vi "Game LaunchPad.vi"() -> ()   [LabVIEW 2011]
uses:
  <vilib>/Utility/miscctls.llb/LVPositionTypeDef.ctl
panel:
  out "life":dbl
  out "showLifeScoreString":string="Life:      Score:"
  out "showTimeString":string="Time:"
  in  "start":bool
  in  "retry":bool
  out "fish":dbl
  out "time":dbl
  in  "stop":bool
  in  "stop 3":bool
  in  "stop 2":bool
  in  "WindowsMediaPlayer 3":refnum<k7>(container)
  in  "WindowsMediaPlayer 2":refnum<k7>(container)
  in  "WindowsMediaPlayer":refnum<k7>(container)
  out "cat sad picture":picture
  out "cat eat picture":picture
  out "win picture":picture
  out "start picture":picture
  out "badfish Array":picture[][](array[picture])
  out "cat picture":picture
  out "cat position[0-9] 2":dbl
  out "carsh? 2":bool
  out "carsh?":bool
  out "cat position[0-9]":dbl
  out "Fish Array":picture[][](array[picture])
  out "CurrentPath":path
  out "background picture":picture
  # "1"
  # "10"
  # "1"
  # "10"
  # "1"
  # "10"
  # "1"
  # "10"
  # "1"
  # "10"
  # "1"
  # "10"
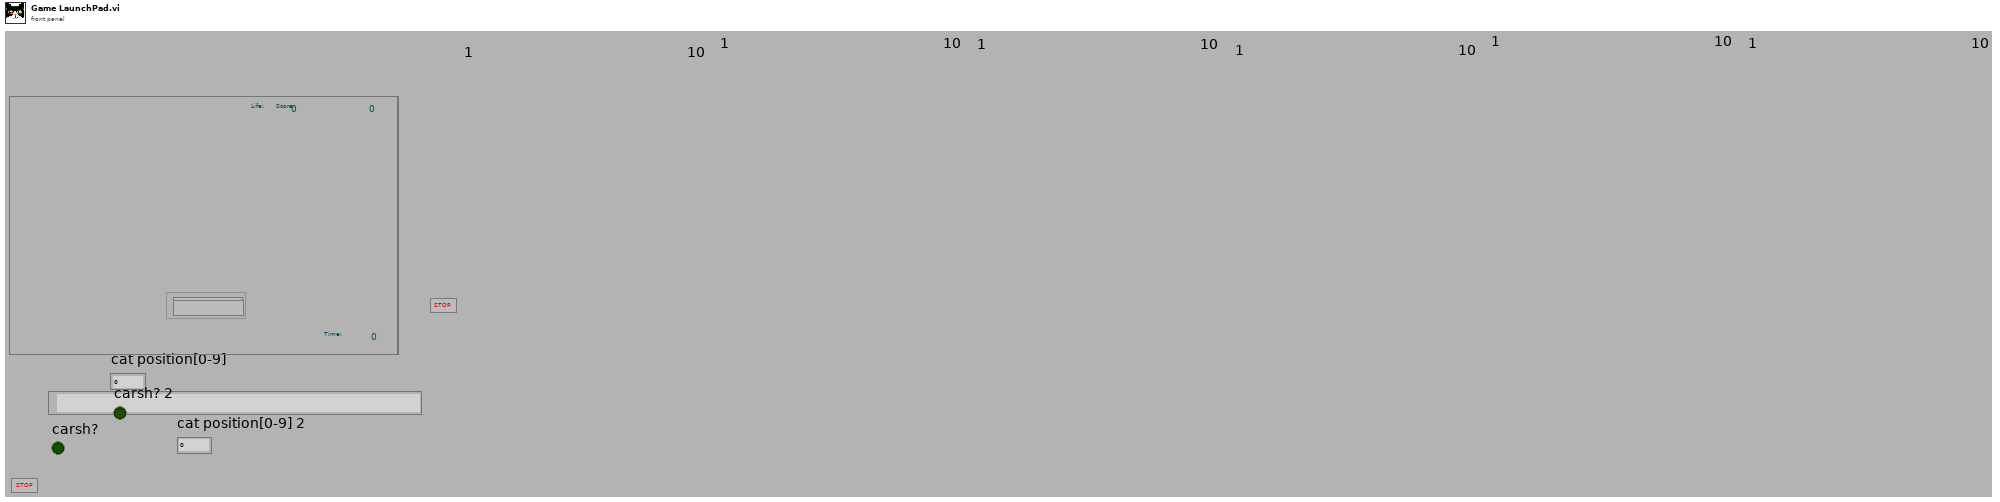
[diagram p1: front panel]
types:
  T1 = enum8{"Enabled", "Disabled", "Disabled and Grayed Out"}
  T2 = typedef "LVPositionTypeDef.ctl" = cluster{"Left":i32, "Top":i32}
  T3 = typedef "imagedata.ctl" = cluster{"image type":i32, "image depth":i32, "image":u8[], "mask":u8[], "colors":u32[], "Rectangle":cluster{"left":i16, "top":i16, "right":i16, "bottom":i16}}
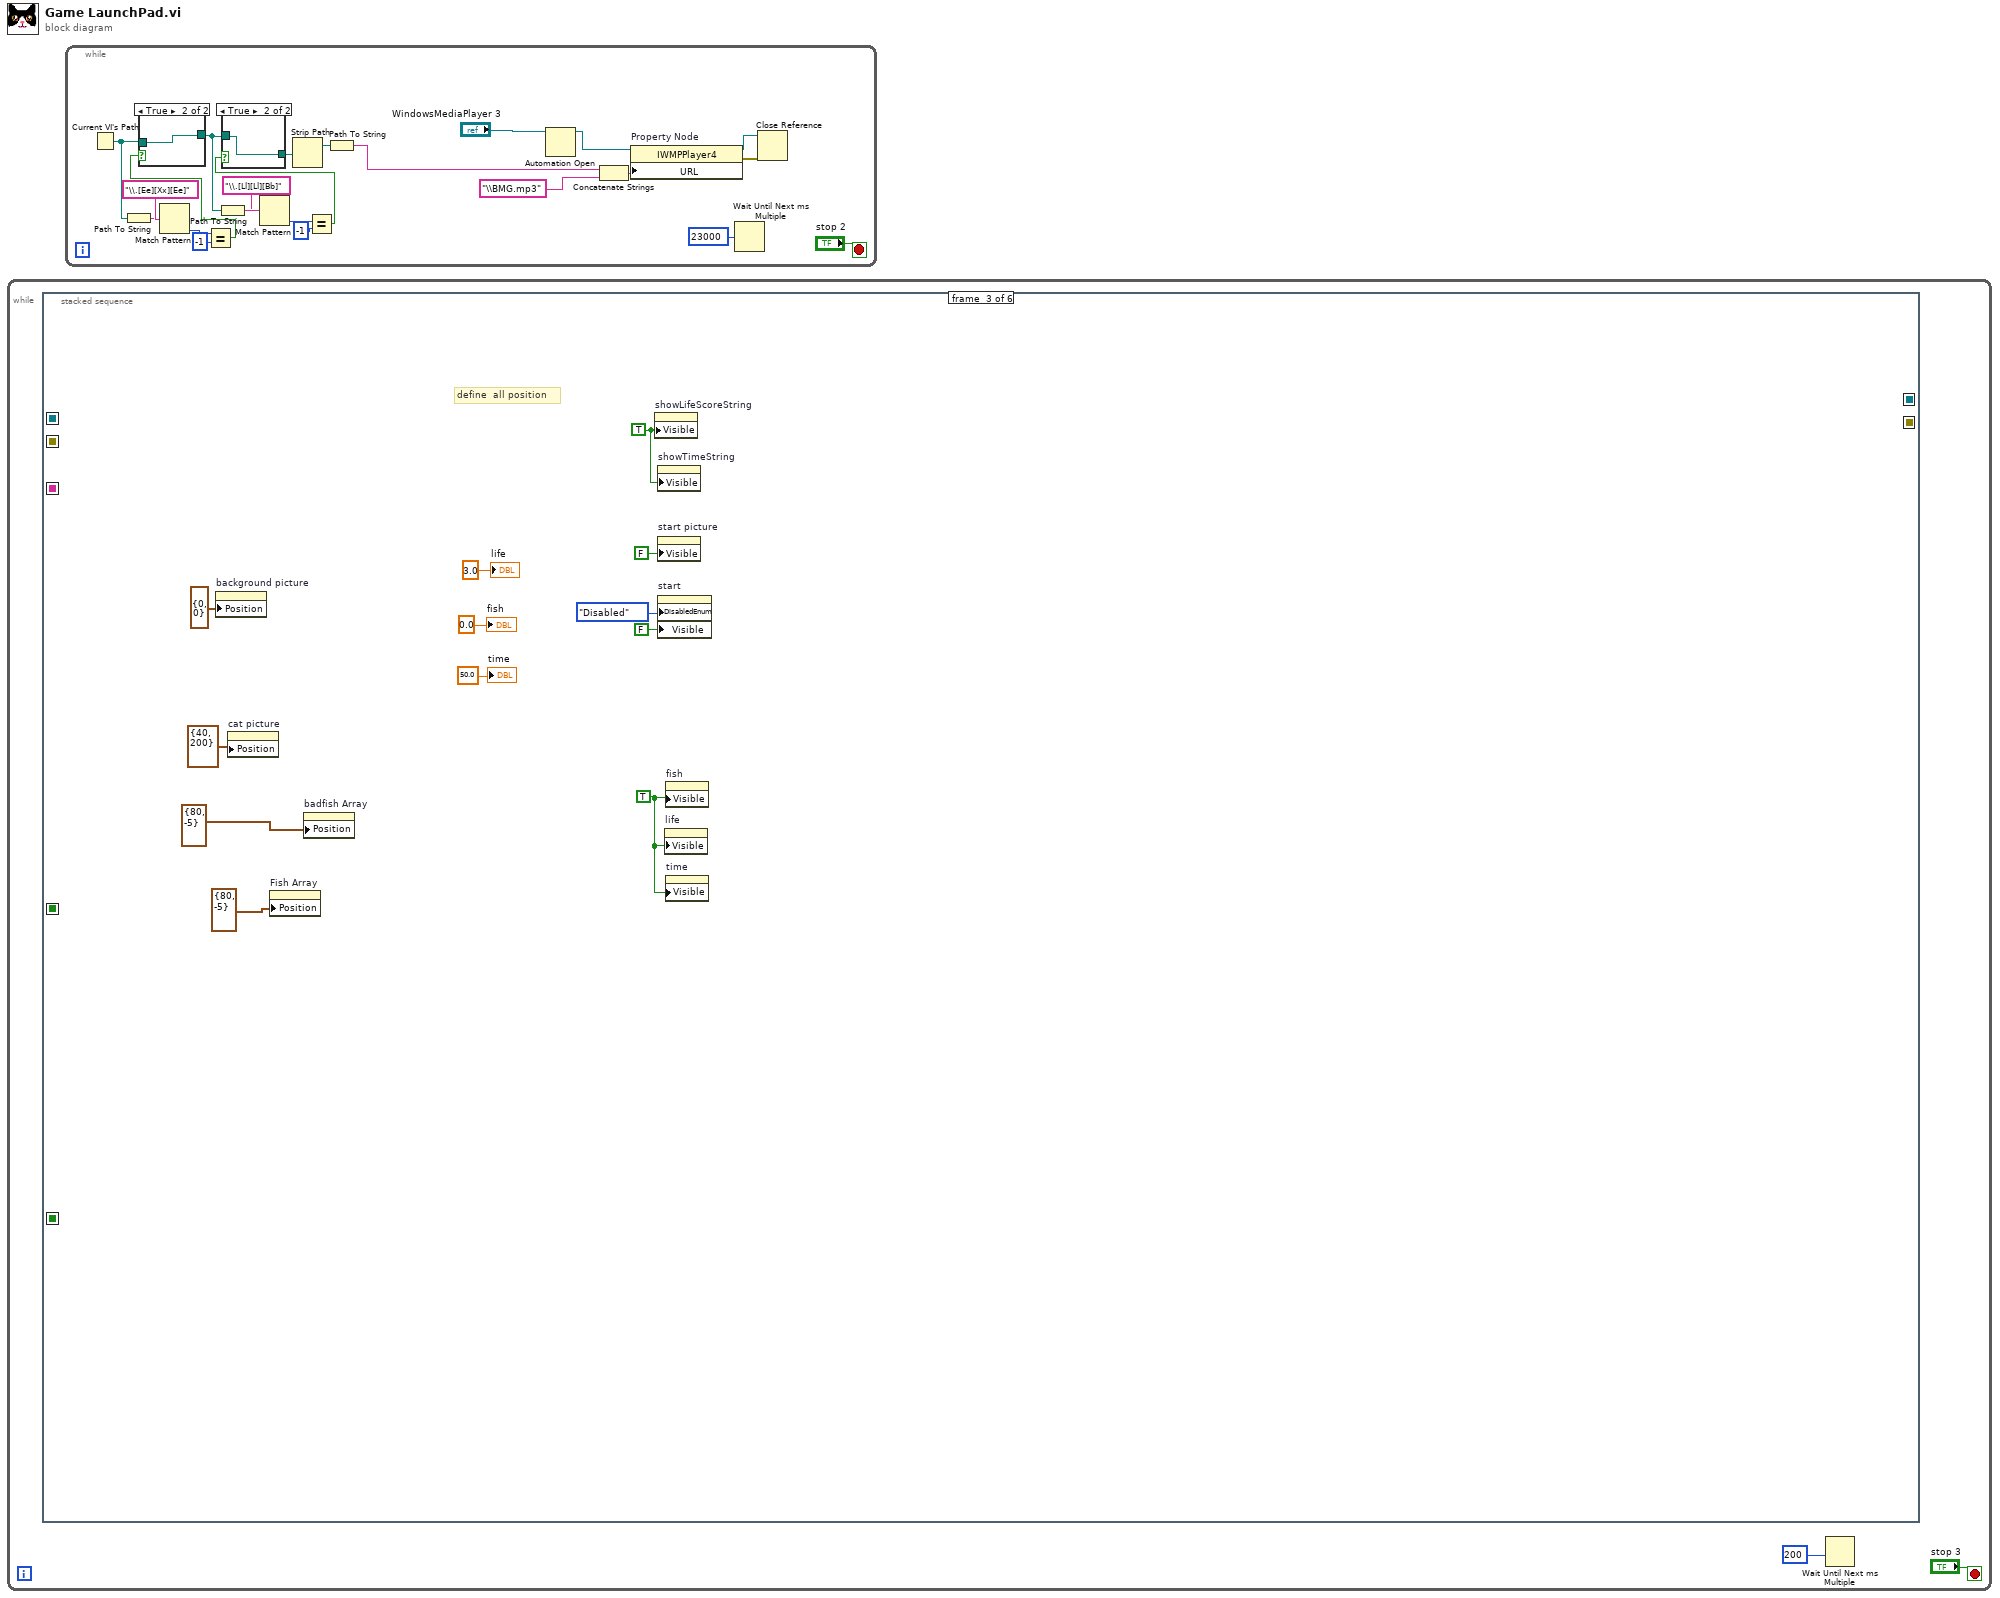
[diagram p0: block diagram]
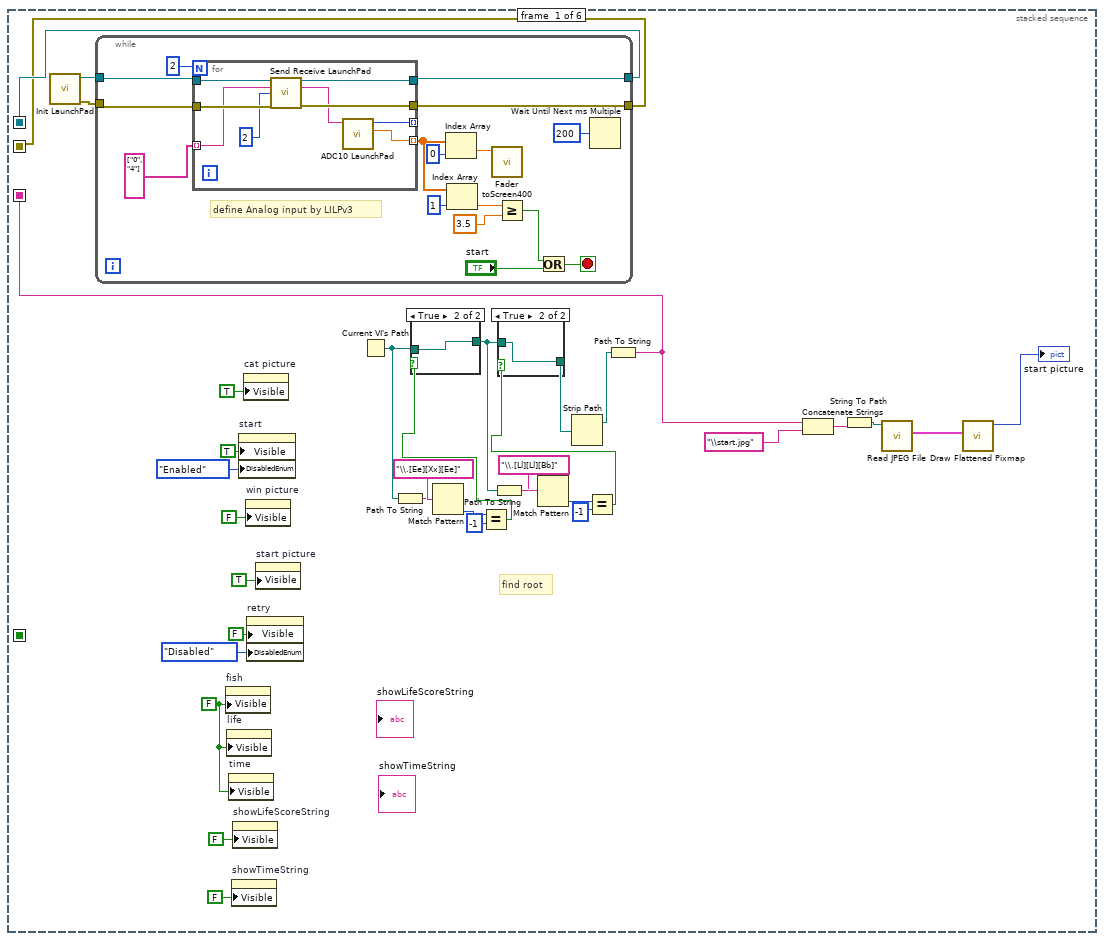
[diagram p2: hidden frame]
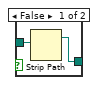
[diagram p3: hidden frame]
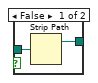
[diagram p4: hidden frame]
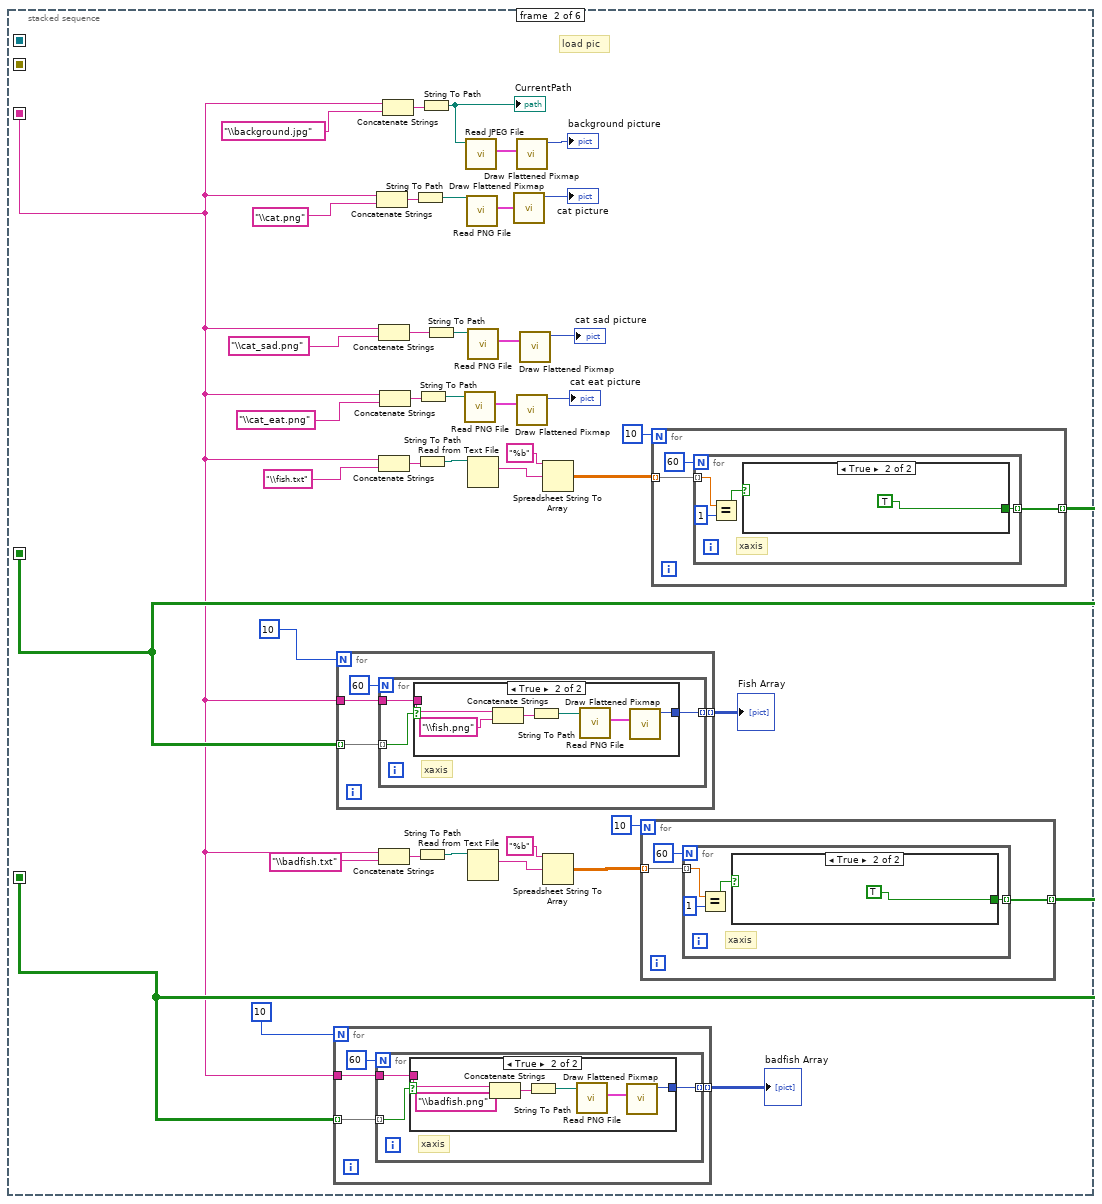
[diagram p5: hidden frame]
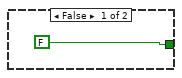
[diagram p6: hidden frame]
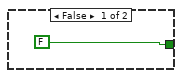
[diagram p7: hidden frame]
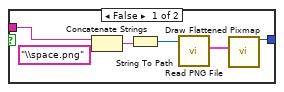
[diagram p8: hidden frame]
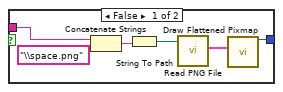
[diagram p9: hidden frame]
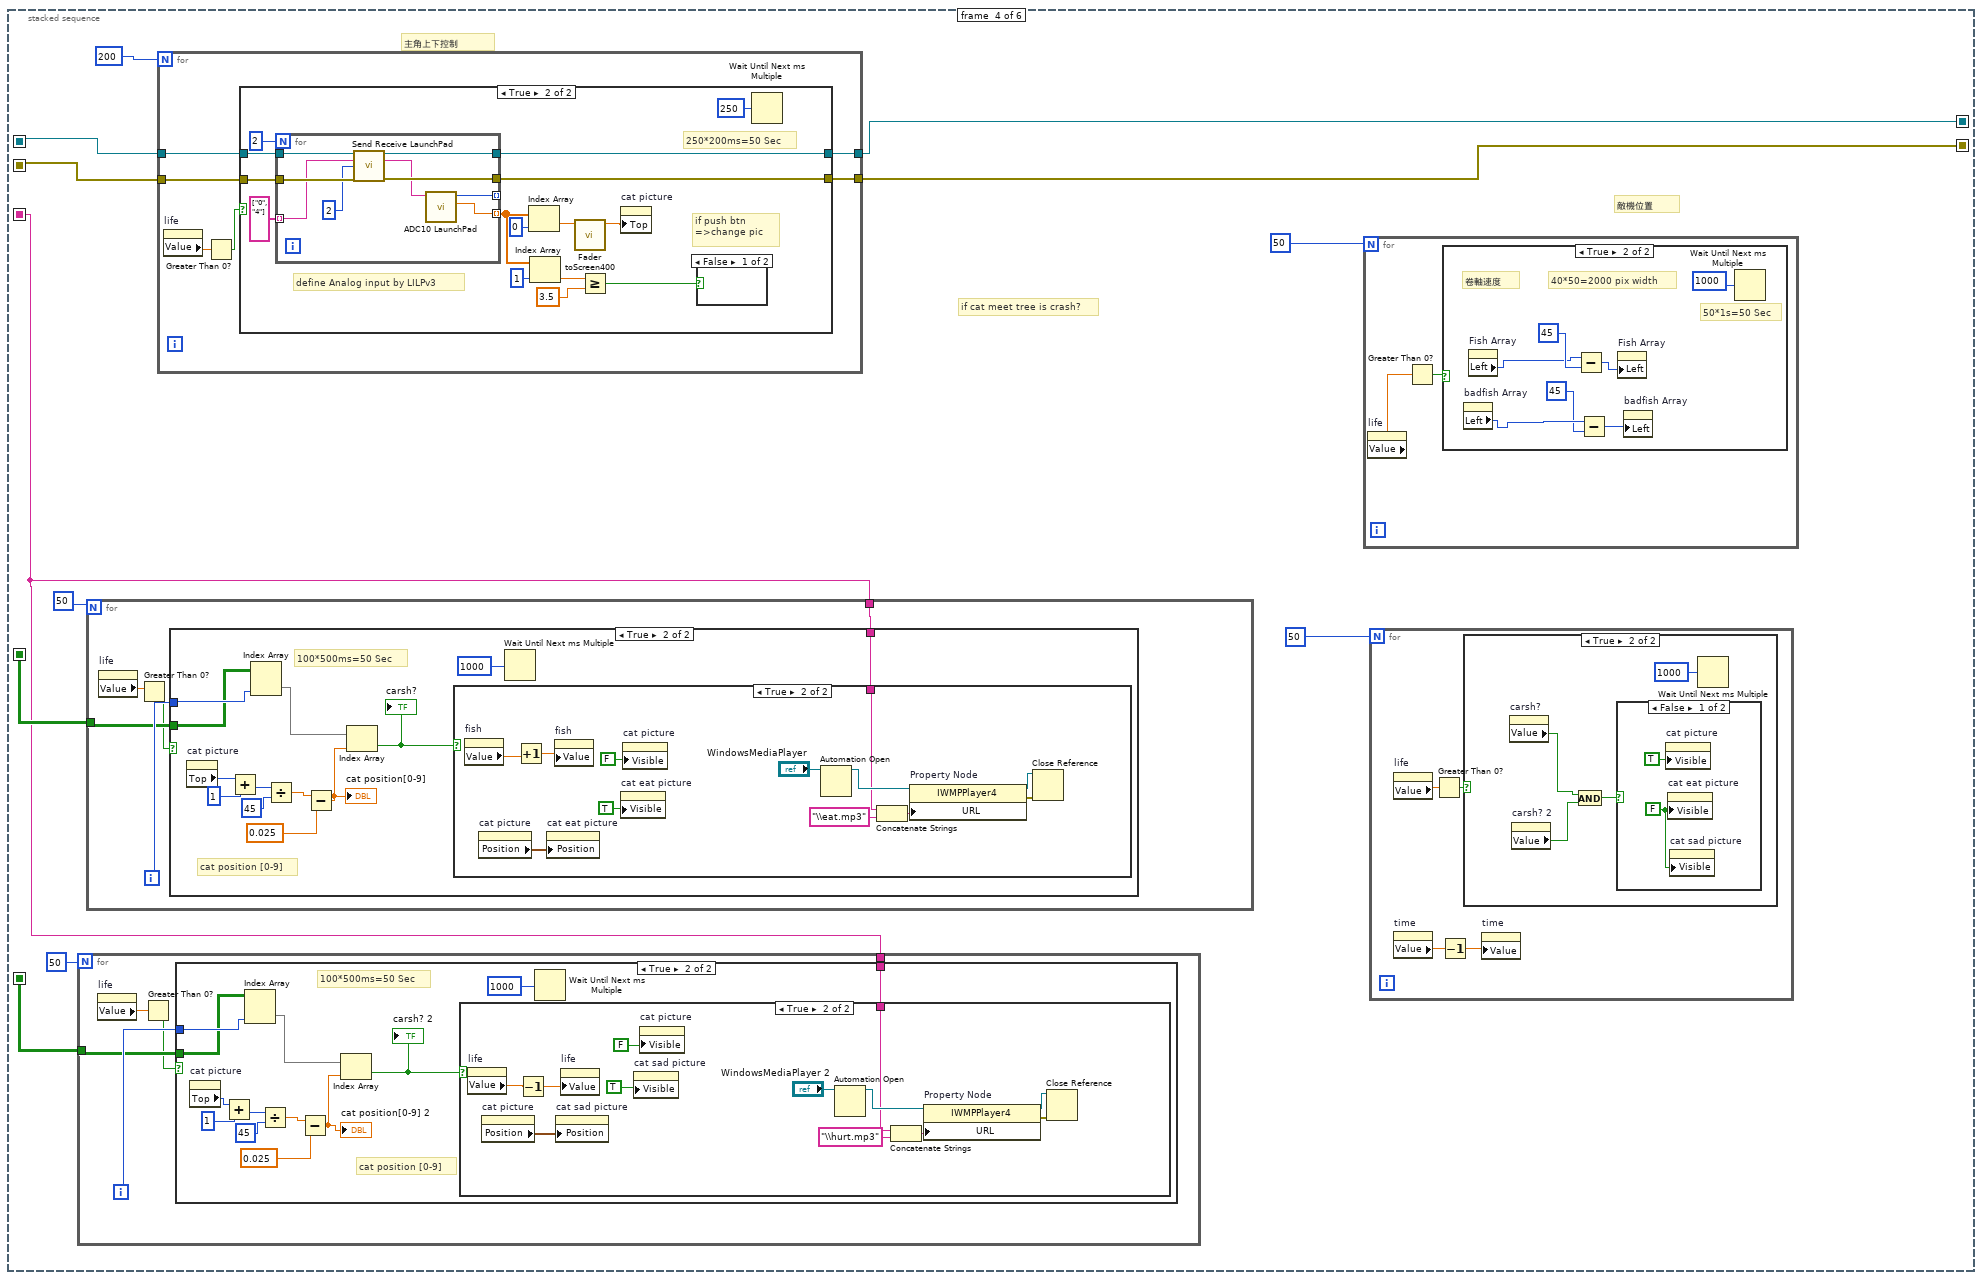
[diagram p10: hidden frame]
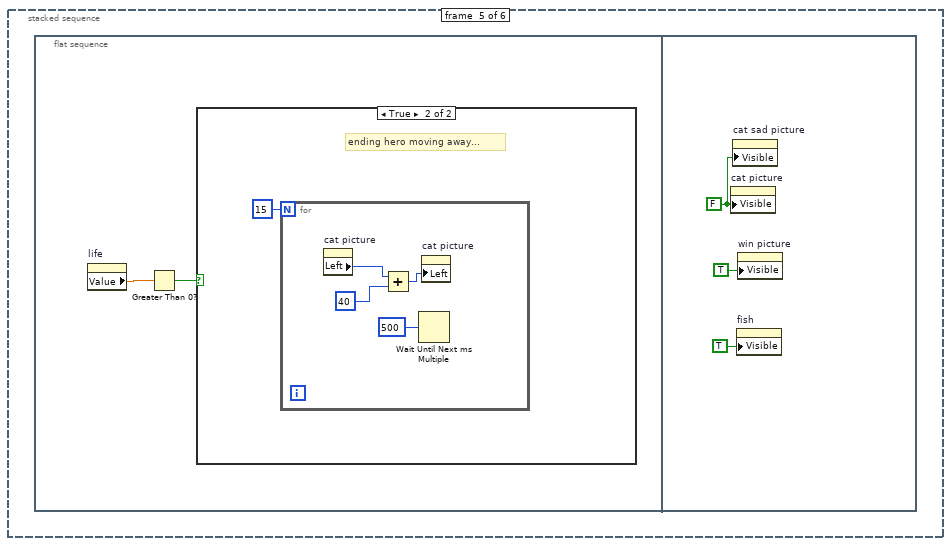
[diagram p20: hidden frame]
diagram:
  n1 = while {
    stop <- "stop 3" stop-if-true
    n2 = stacked-sequence {
      seq-local: [_ w76 _ _ _ _] -> [_ _ _ w184 _ _]
      seq-local: [_ w75 _ _ _ _] -> [_ _ _ w183 _ _]
      seq-local: [w13 _ _ _ _ _] -> [_ w69 _ w179 _ w315]
      seq-local: [w15 _ _ _ _ _] -> [_ _ _ w182 _ _]
      seq-local: [w14 _ _ _ _ _] -> [_ _ _ w181 _ _]
      seq-local: [_ _ _ w178 _ _] -> [_ _ _ _ _ w314]
      seq-local: [_ _ _ w177 _ _] -> [_ _ _ _ _ w313]
      frame #0 {
        w5 = FALSE ("Visible")
        # "find root"
        n3 = call "Init LaunchPad.vi"() -> ("error out"=w16:errorcluster, "VISA resource name out"=w17:refnum<visa-resource-name>)  [unwired: 10 in]
        n4 = while {
          tunnel: w17 -> [w44]
          tunnel: w16 -> [w43]
          tunnel: [w38] -> w15
          tunnel: [w37] -> w14
          stop <- w39 stop-if-true
          # "define Analog input by LILPv3"
          n5 = for {
            N: 2 -> [_]
            tunnel: w44 -> [w61]
            tunnel: [w60] -> w38
            tunnel: [w59] -> w37
            tunnel: w43 -> [w58]
            tunnel: string[] ["0", "4"] -> [w56] mode=indexing
            tunnel: [w54] -> _ mode=indexing
            tunnel: [w53] -> w48 mode=indexing
            n6 = call "Send Receive LaunchPad.vi"("VISA resource"=w61, "write buffer"=w56, "Bytes To Read (0)"=u8 2, "error in"=w58) -> ("VISA resource 2"=w60:refnum<visa-resource-name>, "Read Buffer"=w55:string, "error out"=w59:errorcluster)  [unwired: 9 in]
            n7 = call "ADC10 LaunchPad.vi"("string"=w55) -> ("ADC10 (Volt)"=w53:dbl, "ADCvalue"=w54:u16)  [unwired: 9 in]
          }
          n8 = Index Array(array=w48, index=0) -> (element=w47:dbl)
          n9 = Index Array(array=w48, index=1) -> (element=w45:dbl)
          n10 = call "Fader toScreen400.vi"("Numeric"=w47) -> ()  [unwired: 10 in, 1 out]
          n11 = Greater Or Equal?(x=w45, y=3.5) -> (x >= y?=w41:bool)
          n12 = Or(x=w41, y="start") -> (x .or. y?=w39:bool)
          n13 = Wait Until Next ms Multiple(millisecond multiple=u32 200) -> ()  [unwired: 1 out]
        }
        n14 = property on="fish" class="DigNum (strict)"("Visible"=w5) -> ()  [unwired: 2 in, 2 out]
        n15 = property on="life" class="DigNum (strict)"("Visible"=w5) -> ()  [unwired: 2 in, 2 out]
        n16 = property on="time" class="DigNum (strict)"("Visible"=w5) -> ()  [unwired: 2 in, 2 out]
        n17 = property on="showTimeString" class="Str"("Visible"=FALSE) -> ()  [unwired: 2 in, 2 out]
        n18 = property on="showLifeScoreString" class="Str"("Visible"=FALSE) -> ()  [unwired: 2 in, 2 out]
        n19 = property on="start" class="Bool"("Visible"=TRUE, "DisabledEnum"=T1."Enabled" ("Disabled")) -> ()  [unwired: 2 in, 2 out]
        n20 = property on="cat picture" class="Pict"("Visible"=TRUE) -> ()  [unwired: 2 in, 2 out]
        n21 = property on="win picture" class="Pict"("Visible"=FALSE) -> ()  [unwired: 2 in, 2 out]
        n22 = property on="retry" class="Bool"("Visible"=FALSE, "DisabledEnum"=T1."Disabled" ("Disabled")) -> ()  [unwired: 2 in, 2 out]
        n23 = property on="start picture" class="Pict"("Visible"=TRUE) -> ()  [unwired: 2 in, 2 out]
        n24 = Current VI's Path() -> (path=w27:path)
        n25 = Path To String(path=w27) -> (string=w26:string)
        n26 = Match Pattern(string=w26, regular expression="\\.[Ee][Xx][Ee]") -> (offset past match=w24:i32)  [unwired: 1 in, 3 out]
        n27 = Equal?(x=w24, y=-1) -> (x = y?=w36:bool)
        n28 = case shown="True" w36 {
          tunnel: [w65 w67] -> w33
          tunnel: w27 -> [w66 w67]
          frame False {
            n29 = Strip Path(path=w66) -> (stripped path=w65:path)  [unwired: 1 out]
          }
          frame True {
          }
        }
        n30 = Path To String(path=w33) -> (string=w30:string)
        n31 = Match Pattern(string=w30, regular expression="\\.[Ll][Ll][Bb]") -> (offset past match=w32:i32)  [unwired: 1 in, 3 out]
        n32 = Equal?(x=w32, y=-1) -> (x = y?=w35:bool)
        n33 = case shown="True" w35 {
          tunnel: [w62 w64] -> w34
          tunnel: w33 -> [w63 w64]
          frame False {
            n34 = Strip Path(path=w63) -> (stripped path=w62:path)  [unwired: 1 out]
          }
          frame True {
          }
        }
        n35 = Strip Path(path=w34) -> (stripped path=w23:path)  [unwired: 1 out]
        n36 = Path To String(path=w23) -> (string=w13:string)
        n37 = Concatenate Strings(w13, "\\start.jpg") -> (w19:string)
        n38 = String To Path(string=w19) -> (path=w18:path)
        n39 = call <vilib>:"Read JPEG File.vi"("path to JPEG file"=w18) -> ("image data"=w21:T3)  [unwired: 8 in, 2 out]
        n40 = call <vilib>:"Draw Flattened Pixmap.vi"("image data"=w21) -> ("new picture"=→"start picture":picture)  [unwired: 8 in]
      }
      frame #1 {
        # "load pic"
        n41 = Concatenate Strings(w69, "\\cat.png") -> (w103:string)
        n42 = Concatenate Strings(w69, "\\cat_sad.png") -> (w74:string)
        n43 = Concatenate Strings(w69, "\\fish.txt") -> (w89:string)
        n44 = Concatenate Strings(w69, "\\badfish.txt") -> (w82:string)
        n45 = Concatenate Strings(w69, "\\cat_eat.png") -> (w100:string)
        n46 = Concatenate Strings(w69, "\\background.jpg") -> (w105:string)
        n47 = String To Path(string=w103) -> (path=w97:path)
        n48 = String To Path(string=w89) -> (path=w88:path)
        n49 = String To Path(string=w82) -> (path=w81:path)
        n50 = String To Path(string=w100) -> (path=w95:path)
        n51 = String To Path(string=w105) -> (path=w104:path)
        "CurrentPath" <- w104
        n52 = String To Path(string=w74) -> (path=w71:path)
        n53 = call <vilib>:"Read PNG File.vi"("path to PNG file"=w95) -> ("image data"=w94:T3)  [unwired: 8 in, 2 out]
        n54 = call <vilib>:"Read JPEG File.vi"("path to JPEG file"=w104) -> ("image data"=w107:T3)  [unwired: 8 in, 2 out]
        n55 = call <vilib>:"Read PNG File.vi"("path to PNG file"=w97) -> ("image data"=w96:T3)  [unwired: 8 in, 2 out]
        n56 = call <vilib>:"Read PNG File.vi"("path to PNG file"=w71) -> ("image data"=w70:T3)  [unwired: 8 in, 2 out]
        n57 = Read from Text File(file (use dialog)=w88) -> (text=w87:string)  [unwired: 3 in, 3 out]
        n58 = Read from Text File(file (use dialog)=w81) -> (text=w80:string)  [unwired: 3 in, 3 out]
        n59 = call <vilib>:"Draw Flattened Pixmap.vi"("image data"=w96) -> ("new picture"=→"cat picture":picture)  [unwired: 8 in]
        n60 = call <vilib>:"Draw Flattened Pixmap.vi"("image data"=w107) -> ("new picture"=→"background picture":picture)  [unwired: 8 in]
        n61 = call <vilib>:"Draw Flattened Pixmap.vi"("image data"=w94) -> ("new picture"=→"cat eat picture":picture)  [unwired: 8 in]
        n62 = call <vilib>:"Draw Flattened Pixmap.vi"("image data"=w70) -> ("new picture"=→"cat sad picture":picture)  [unwired: 8 in]
        n63 = Spreadsheet String To Array(format string="%b", spreadsheet string=w87) -> (array=w84:dbl[][])  [unwired: 2 in]
        n64 = Spreadsheet String To Array(format string="%b", spreadsheet string=w80) -> (array=w77:dbl[][])  [unwired: 2 in]
        n65 = for {
          N: 10 -> [_]
          tunnel: w77 -> [w111] mode=indexing
          tunnel: [w109] -> w75 mode=indexing
          n66 = for {
            N: 60 -> [_]
            tunnel: w111 -> [w112] mode=indexing
            tunnel: [w113] -> w109 mode=indexing
            # "xaxis"
            n67 = Equal?(x=w112, y=u16 1) -> (x = y?=w114:bool)
            n68 = case shown="True" w114 {
              tunnel: [FALSE TRUE] -> w113
              frame False {
              }
              frame True {
              }
            }
          }
        }
        n69 = for {
          N: 10 -> [_]
          tunnel: w69 -> [w130]
          tunnel: [w129] -> w68 mode=indexing
          tunnel: w75 -> [w128] mode=indexing
          n70 = for {
            N: 60 -> [_]
            tunnel: w130 -> [w133]
            tunnel: [w132] -> w129 mode=indexing
            tunnel: w128 -> [w131] mode=indexing
            # "xaxis"
            n71 = case shown="True" w131 {
              tunnel: w133 -> [w135 w141]
              tunnel: [w134 w140] -> w132
              frame False {
                n72 = Concatenate Strings(w135, "\\space.png") -> (w136:string)
                n73 = String To Path(string=w136) -> (path=w138:path)
                n74 = call <vilib>:"Read PNG File.vi"("path to PNG file"=w138) -> ("image data"=w139:T3)  [unwired: 8 in, 2 out]
                n75 = call <vilib>:"Draw Flattened Pixmap.vi"("image data"=w139) -> ("new picture"=w134:picture)  [unwired: 8 in]
              }
              frame True {
                n76 = Concatenate Strings(w141, "\\badfish.png") -> (w142:string)
                n77 = String To Path(string=w142) -> (path=w144:path)
                n78 = call <vilib>:"Read PNG File.vi"("path to PNG file"=w144) -> ("image data"=w145:T3)  [unwired: 8 in, 2 out]
                n79 = call <vilib>:"Draw Flattened Pixmap.vi"("image data"=w145) -> ("new picture"=w140:picture)  [unwired: 8 in]
              }
            }
          }
        }
        "badfish Array" <- w68
        n80 = for {
          N: 10 -> [_]
          tunnel: w84 -> [w120] mode=indexing
          tunnel: [w118] -> w76 mode=indexing
          n81 = for {
            N: 60 -> [_]
            tunnel: w120 -> [w121] mode=indexing
            tunnel: [w122] -> w118 mode=indexing
            # "xaxis"
            n82 = Equal?(x=w121, y=u16 1) -> (x = y?=w123:bool)
            n83 = case shown="True" w123 {
              tunnel: [FALSE TRUE] -> w122
              frame False {
              }
              frame True {
              }
            }
          }
        }
        n84 = for {
          N: 10 -> [_]
          tunnel: w69 -> [w149]
          tunnel: [w148] -> w92 mode=indexing
          tunnel: w76 -> [w147] mode=indexing
          n85 = for {
            N: 60 -> [_]
            tunnel: w149 -> [w152]
            tunnel: [w151] -> w148 mode=indexing
            tunnel: w147 -> [w150] mode=indexing
            # "xaxis"
            n86 = case shown="True" w150 {
              tunnel: w152 -> [w154 w160]
              tunnel: [w153 w159] -> w151
              frame False {
                n87 = Concatenate Strings(w154, "\\space.png") -> (w155:string)
                n88 = String To Path(string=w155) -> (path=w157:path)
                n89 = call <vilib>:"Read PNG File.vi"("path to PNG file"=w157) -> ("image data"=w158:T3)  [unwired: 8 in, 2 out]
                n90 = call <vilib>:"Draw Flattened Pixmap.vi"("image data"=w158) -> ("new picture"=w153:picture)  [unwired: 8 in]
              }
              frame True {
                n91 = Concatenate Strings(w160, "\\fish.png") -> (w161:string)
                n92 = String To Path(string=w161) -> (path=w163:path)
                n93 = call <vilib>:"Read PNG File.vi"("path to PNG file"=w163) -> ("image data"=w164:T3)  [unwired: 8 in, 2 out]
                n94 = call <vilib>:"Draw Flattened Pixmap.vi"("image data"=w164) -> ("new picture"=w159:picture)  [unwired: 8 in]
              }
            }
          }
        }
        "Fish Array" <- w92
      }
      frame #2 {
        w166 = TRUE ("Visible")
        w165 = TRUE ("Visible")
        # "define  all position"
        n95 = property on="background picture" class="Pict"("Position"=T2 {"Left"=0, "Top"=0}) -> ()  [unwired: 2 in, 2 out]
        n96 = property on="cat picture" class="Pict"("Position"=T2 {"Left"=40, "Top"=200}) -> ()  [unwired: 2 in, 2 out]
        n97 = property on="Fish Array" class="Arr (strict)"("Position"=T2 {"Left"=80, "Top"=-5}) -> ()  [unwired: 2 in, 2 out]
        n98 = property on="badfish Array" class="Arr (strict)"("Position"=T2 {"Left"=80, "Top"=-5}) -> ()  [unwired: 2 in, 2 out]
        n99 = property on="showLifeScoreString" class="Str"("Visible"=w166) -> ()  [unwired: 2 in, 2 out]
        n100 = property on="showTimeString" class="Str"("Visible"=w166) -> ()  [unwired: 2 in, 2 out]
        n101 = property on="start picture" class="Pict"("Visible"=FALSE) -> ()  [unwired: 2 in, 2 out]
        n102 = property on="start" class="Bool"("DisabledEnum"=T1."Disabled" ("Disabled"), "Visible"=FALSE) -> ()  [unwired: 2 in, 2 out]
        n103 = property on="life" class="DigNum (strict)"("Visible"=w165) -> ()  [unwired: 2 in, 2 out]
        n104 = property on="fish" class="DigNum (strict)"("Visible"=w165) -> ()  [unwired: 2 in, 2 out]
        n105 = property on="time" class="DigNum (strict)"("Visible"=w165) -> ()  [unwired: 2 in, 2 out]
        "life" <- 3.0 ("Numeric")
        "fish" <- 0.0 ("Numeric")
        "time" <- 50.0 ("time")
      }
      frame #3 {
        # "敵機位置"
        # "主角上下控制"
        # "if cat meet tree is crash?"
        n106 = for {
          N: 50 -> [_]
          tunnel: w183 -> [w202]
          tunnel: w179 -> [w199]
          i -> [w203]
          n107 = property on="life" class="DigNum (strict)"() -> ("Value"=w201:dbl)  [unwired: 2 in, 2 out]
          n108 = Greater Than 0?(x=w201) -> (x > 0?=w200:bool)
          n109 = case shown="True" w200 {
            tunnel: w203 -> [_ w215]
            tunnel: w202 -> [_ w207]
            tunnel: w199 -> [_ w204]
            frame False {
            }
            frame True {
              # "cat position [0-9]"
              # "100*500ms=50 Sec"
              n110 = property on="cat picture" class="Pict"() -> ("Top"=w205:i32)  [unwired: 2 in, 2 out]
              n111 = Add(x=w205, y=1) -> (x+y=w213:i32)
              n112 = Index Array(array=w207, index (col)=w215) -> (element=w209:bool[])  [unwired: 1 in]
              n113 = Divide(x=w213, y=45) -> (x/y=w211:dbl)
              n114 = Subtract(x=w211, y=0.025) -> (x-y=w208:dbl)
              "cat position[0-9] 2" <- w208
              n115 = Index Array(array=w209, index=w208) -> (element=w206:bool)
              "carsh? 2" <- w206
              n116 = case shown="True" w206 {
                tunnel: w204 -> [_ w218]
                frame False {
                }
                frame True {
                  n117 = property on="life" class="DigNum (strict)"() -> ("Value"=w228:dbl)  [unwired: 2 in, 2 out]
                  n118 = property on="cat picture" class="Pict"() -> ("Position"=w226:T2)  [unwired: 2 in, 2 out]
                  n119 = Decrement(x=w228) -> (x-1=w227:dbl)
                  n120 = property on="cat sad picture" class="Pict"("Position"=w226) -> ()  [unwired: 2 in, 2 out]
                  n121 = property on="life" class="DigNum (strict)"("Value"=w227) -> ()  [unwired: 2 in, 2 out]
                  n122 = property on="cat sad picture" class="Pict"("Visible"=TRUE) -> ()  [unwired: 2 in, 2 out]
                  n123 = property on="cat picture" class="Pict"("Visible"=FALSE) -> ()  [unwired: 2 in, 2 out]
                  n124 = Automation Open(Automation Refnum="WindowsMediaPlayer 2") -> (Automation Refnum=w223:refnum<k7>)  [unwired: 1 in, 3 out]
                  n125 = Concatenate Strings(w218, "\\hurt.mp3" ("string")) -> (w217:string)
                  n126 = property on="Property Node" class="IWMPPlayer4"(reference=w223, "URL"=w217) -> (reference out=w221:refnum<k7>, error out=w220:errorcluster)  [unwired: 1 in]
                  n127 = Close Reference(reference=w221, error in (no error)=w220) -> ()  [unwired: 1 out]
                }
              }
              n128 = Wait Until Next ms Multiple(millisecond multiple=u32 1000 ("millisecond timer value")) -> ()  [unwired: 1 out]
            }
          }
        }
        n129 = for {
          N: 50 -> [_]
          tunnel: w184 -> [w232]
          tunnel: w179 -> [w229]
          i -> [w233]
          n130 = property on="life" class="DigNum (strict)"() -> ("Value"=w231:dbl)  [unwired: 2 in, 2 out]
          n131 = Greater Than 0?(x=w231) -> (x > 0?=w230:bool)
          n132 = case shown="True" w230 {
            tunnel: w233 -> [_ w245]
            tunnel: w232 -> [_ w236]
            tunnel: w229 -> [_ w234]
            frame False {
            }
            frame True {
              # "cat position [0-9]"
              # "100*500ms=50 Sec"
              n133 = property on="cat picture" class="Pict"() -> ("Top"=w244:i32)  [unwired: 2 in, 2 out]
              n134 = Add(x=w244, y=1) -> (x+y=w242:i32)
              n135 = Index Array(array=w236, index (col)=w245) -> (element=w238:bool[])  [unwired: 1 in]
              n136 = Divide(x=w242, y=45) -> (x/y=w240:dbl)
              n137 = Subtract(x=w240, y=0.025) -> (x-y=w237:dbl)
              "cat position[0-9]" <- w237
              n138 = Index Array(array=w238, index=w237) -> (element=w235:bool)
              "carsh?" <- w235
              n139 = case shown="True" w235 {
                tunnel: w234 -> [_ w249]
                frame False {
                }
                frame True {
                  n140 = property on="fish" class="DigNum (strict)"() -> ("Value"=w258:dbl)  [unwired: 2 in, 2 out]
                  n141 = property on="cat picture" class="Pict"() -> ("Position"=w254:T2)  [unwired: 2 in, 2 out]
                  n142 = Increment(x=w258) -> (x+1=w257:dbl)
                  n143 = property on="cat eat picture" class="Pict"("Position"=w254) -> ()  [unwired: 2 in, 2 out]
                  n144 = property on="fish" class="DigNum (strict)"("Value"=w257) -> ()  [unwired: 2 in, 2 out]
                  n145 = property on="cat eat picture" class="Pict"("Visible"=TRUE) -> ()  [unwired: 2 in, 2 out]
                  n146 = property on="cat picture" class="Pict"("Visible"=FALSE) -> ()  [unwired: 2 in, 2 out]
                  n147 = Automation Open(Automation Refnum="WindowsMediaPlayer") -> (Automation Refnum=w253:refnum<k7>)  [unwired: 1 in, 3 out]
                  n148 = Concatenate Strings(w249, "\\eat.mp3" ("string")) -> (w248:string)
                  n149 = property on="Property Node" class="IWMPPlayer4"(reference=w253, "URL"=w248) -> (reference out=w251:refnum<k7>, error out=w250:errorcluster)  [unwired: 1 in]
                  n150 = Close Reference(reference=w251, error in (no error)=w250) -> ()  [unwired: 1 out]
                }
              }
              n151 = Wait Until Next ms Multiple(millisecond multiple=u32 1000 ("millisecond timer value")) -> ()  [unwired: 1 out]
            }
          }
        }
        n152 = for {
          N: 200 -> [_]
          tunnel: w182 -> [w264]
          tunnel: w181 -> [w263]
          tunnel: [w262] -> w178
          tunnel: [w261] -> w177
          n153 = property on="life" class="DigNum (strict)"() -> ("Value"=w260:dbl)  [unwired: 2 in, 2 out]
          n154 = Greater Than 0?(x=w260) -> (x > 0?=w259:bool)
          n155 = case shown="True" w259 {
            tunnel: w264 -> [w266 w281]
            tunnel: w263 -> [w265 w280]
            tunnel: [w266 w278] -> w262
            tunnel: [w265 w277] -> w261
            frame False {
            }
            frame True {
              # "define Analog input by LILPv3"
              # "if push btn \n=>change pic"
              # "250*200ms=50 Sec"
              n156 = for {
                N: 2 -> [_]
                tunnel: w281 -> [w290]
                tunnel: [w289] -> w278
                tunnel: [w288] -> w277
                tunnel: w280 -> [w287]
                tunnel: string[] ["0", "4"] -> [w285] mode=indexing
                tunnel: [w283] -> _ mode=indexing
                tunnel: [w282] -> w273 mode=indexing
                n157 = call "Send Receive LaunchPad.vi"("VISA resource"=w290, "write buffer"=w285, "Bytes To Read (0)"=u8 2, "error in"=w287) -> ("VISA resource 2"=w289:refnum<visa-resource-name>, "Read Buffer"=w284:string, "error out"=w288:errorcluster)  [unwired: 9 in]
                n158 = call "ADC10 LaunchPad.vi"("string"=w284) -> ("ADC10 (Volt)"=w282:dbl, "ADCvalue"=w283:u16)  [unwired: 9 in]
              }
              n159 = Index Array(array=w273, index=0) -> (element=w271:dbl)
              n160 = Index Array(array=w273, index=1) -> (element=w268:dbl)
              n161 = call "Fader toScreen400.vi"("Numeric"=w271) -> ("Numeric 2"=w270:dbl)  [unwired: 10 in]
              n162 = Greater Or Equal?(x=w268, y=3.5) -> (x >= y?=w267:bool)
              n163 = property on="cat picture" class="Pict"("Top"=w270) -> ()  [unwired: 2 in, 2 out]
              n164 = case shown="False" w267 {
                frame False {
                }
                frame True {
                }
              }
              n165 = Wait Until Next ms Multiple(millisecond multiple=u32 250) -> ()  [unwired: 1 out]
            }
          }
        }
        n166 = for {
          N: 50 -> [_]
          n167 = property on="life" class="DigNum (strict)"() -> ("Value"=w291:dbl)  [unwired: 2 in, 2 out]
          n168 = Greater Than 0?(x=w291) -> (x > 0?=w292:bool)
          n169 = case shown="True" w292 {
            frame False {
            }
            frame True {
              # "50*1s=50 Sec"
              # "40*50=2000 pix width"
              # "卷軸速度"
              n170 = property on="badfish Array" class="Arr (strict)"() -> ("Left"=w295:i32)  [unwired: 2 in, 2 out]
              n171 = property on="Fish Array" class="Arr (strict)"() -> ("Left"=w297:i32)  [unwired: 2 in, 2 out]
              n172 = Subtract(x=w297, y=45) -> (x-y=w296:i32)
              n173 = Subtract(x=w295, y=45) -> (x-y=w294:i32)
              n174 = property on="Fish Array" class="Arr (strict)"("Left"=w296) -> ()  [unwired: 2 in, 2 out]
              n175 = property on="badfish Array" class="Arr (strict)"("Left"=w294) -> ()  [unwired: 2 in, 2 out]
              n176 = Wait Until Next ms Multiple(millisecond multiple=u32 1000 ("millisecond timer value")) -> ()  [unwired: 1 out]
            }
          }
        }
        n177 = for {
          N: 50 -> [_]
          n178 = property on="life" class="DigNum (strict)"() -> ("Value"=w191:dbl)  [unwired: 2 in, 2 out]
          n179 = property on="time" class="DigNum (strict)"() -> ("Value"=w190:dbl)  [unwired: 2 in, 2 out]
          n180 = Greater Than 0?(x=w191) -> (x > 0?=w192:bool)
          n181 = Decrement(x=w190) -> (x-1=w189:dbl)
          n182 = case shown="True" w192 {
            frame False {
            }
            frame True {
              n183 = property on="carsh?" class="Bool (strict)"() -> ("Value"=w196:bool)  [unwired: 2 in, 2 out]
              n184 = property on="carsh? 2" class="Bool (strict)"() -> ("Value"=w195:bool)  [unwired: 2 in, 2 out]
              n185 = And(x=w196, y=w195) -> (x .and. y?=w194:bool)
              n186 = case shown="False" w194 {
                frame False {
                  w197 = FALSE ("Visible")
                  n187 = property on="cat picture" class="Pict"("Visible"=TRUE) -> ()  [unwired: 2 in, 2 out]
                  n188 = property on="cat eat picture" class="Pict"("Visible"=w197) -> ()  [unwired: 2 in, 2 out]
                  n189 = property on="cat sad picture" class="Pict"("Visible"=w197) -> ()  [unwired: 2 in, 2 out]
                }
                frame True {
                }
              }
              n190 = Wait Until Next ms Multiple(millisecond multiple=u32 1000) -> ()  [unwired: 1 out]
            }
          }
          n191 = property on="time" class="DigNum (strict)"("Value"=w189) -> ()  [unwired: 2 in, 2 out]
        }
      }
      frame #4 {
        n192 = flat-sequence {
          frame #0 {
            n193 = property on="life" class="DigNum (strict)"() -> ("Value"=w301:dbl)  [unwired: 2 in, 2 out]
            n194 = Greater Than 0?(x=w301) -> (x > 0?=w300:bool)
            n195 = case shown="True" w300 {
              frame False {
                # "skip"
              }
              frame True {
                # "ending hero moving away..."
                n196 = for {
                  N: 15 -> [_]
                  n197 = property on="cat picture" class="Pict"() -> ("Left"=w306:i32)  [unwired: 2 in, 2 out]
                  n198 = Add(x=w306, y=40) -> (x+y=w304:i32)
                  n199 = Wait Until Next ms Multiple(millisecond multiple=u32 500 ("millisecond timer value")) -> ()  [unwired: 1 out]
                  n200 = property on="cat picture" class="Pict"("Left"=w304) -> ()  [unwired: 2 in, 2 out]
                }
              }
            }
          }
          frame #1 {
            w307 = FALSE ("Visible")
            n201 = property on="cat picture" class="Pict"("Visible"=w307) -> ()  [unwired: 2 in, 2 out]
            n202 = property on="cat sad picture" class="Pict"("Visible"=w307) -> ()  [unwired: 2 in, 2 out]
            n203 = property on="fish" class="DigNum (strict)"("Visible"=TRUE) -> ()  [unwired: 2 in, 2 out]
            n204 = property on="win picture" class="Pict"("Visible"=TRUE) -> ()  [unwired: 2 in, 2 out]
          }
        }
      }
      frame #5 {
        # "play end message and close game"
        n205 = flat-sequence {
          tunnel: w315 -> [w321]
          tunnel: w314 -> [w317]
          tunnel: w313 -> [w316]
          tunnel: [w318] -> w312
          tunnel: [w317] -> w311
          tunnel: [w316] -> w310
          tunnel: w312 -> [w333]
          tunnel: w311 -> [w332]
          tunnel: w310 -> [w331]
          frame #0 {
            n206 = property on="life" class="DigNum (strict)"() -> ("Value"=w320:dbl)  [unwired: 2 in, 2 out]
            n207 = Less Or Equal To 0?(x=w320) -> (x <= 0?=w318:bool)
            n208 = case shown="True" w318 {
              tunnel: ["\\win.jpg" "\\lose.jpg"] -> w319
              frame False {
              }
              frame True {
                n209 = property on="retry" class="Bool"("Visible"=TRUE, "DisabledEnum"=T1."Enabled" ("Disabled")) -> ()  [unwired: 2 in, 2 out]
              }
            }
            n210 = Concatenate Strings(w321, w319) -> (w323:string)
            n211 = String To Path(string=w323) -> (path=w322:path)
            n212 = call <vilib>:"Read JPEG File.vi"("path to JPEG file"=w322) -> ("image data"=w324:T3)  [unwired: 8 in, 2 out]
            n213 = call <vilib>:"Draw Flattened Pixmap.vi"("image data"=w324) -> ("new picture"=→"win picture":picture)  [unwired: 8 in]
          }
          frame #1 {
            # "show lose / win and inf loop"
            n214 = case shown="True" w333 {
              tunnel: w332 -> [_ w337]
              tunnel: w331 -> [_ w336]
              frame False {
                n215 = while {
                  stop <- "stop" stop-if-true
                  n216 = Wait Until Next ms Multiple(millisecond multiple=u32 500 ("millisecond timer value")) -> ()  [unwired: 1 out]
                }
              }
              frame True {
                # "lose and retry"
                n217 = while {
                  tunnel: w337 -> [w347]
                  tunnel: [w342] -> w339
                  tunnel: [w341] -> w338
                  tunnel: w336 -> [w340]
                  stop <- w343 stop-if-true
                  # "define Analog input by LILPv3"
                  n218 = for {
                    N: 2 -> [_]
                    tunnel: w347 -> [w364]
                    tunnel: [w363] -> w342
                    tunnel: [w362] -> w341
                    tunnel: w340 -> [w361]
                    tunnel: string[] ["0", "4"] -> [w359] mode=indexing
                    tunnel: [w357] -> _ mode=indexing
                    tunnel: [w356] -> w351 mode=indexing
                    n219 = call "Send Receive LaunchPad.vi"("VISA resource"=w364, "write buffer"=w359, "Bytes To Read (0)"=u8 2, "error in"=w361) -> ("VISA resource 2"=w363:refnum<visa-resource-name>, "Read Buffer"=w358:string, "error out"=w362:errorcluster)  [unwired: 9 in]
                    n220 = call "ADC10 LaunchPad.vi"("string"=w358) -> ("ADC10 (Volt)"=w356:dbl, "ADCvalue"=w357:u16)  [unwired: 9 in]
                  }
                  n221 = Index Array(array=w351, index=0) -> (element=w350:dbl)
                  n222 = Index Array(array=w351, index=1) -> (element=w348:dbl)
                  n223 = call "Fader toScreen400.vi"("Numeric"=w350) -> ()  [unwired: 10 in, 1 out]
                  n224 = Greater Or Equal?(x=w348, y=3.5) -> (x >= y?=w345:bool)
                  n225 = Or(x=w345, y="retry") -> (x .or. y?=w343:bool)
                  n226 = Wait Until Next ms Multiple(millisecond multiple=u32 200) -> ()  [unwired: 1 out]
                }
                n227 = call "Close LaunchPad.vi"("VISA resource name"=w339, "error in"=w338) -> ()  [unwired: 13 in, 1 out]
              }
            }
            n228 = property on="life" class="DigNum (strict)"("Visible"=TRUE) -> ()  [unwired: 2 in, 2 out]
          }
        }
      }
    }
    n229 = Wait Until Next ms Multiple(millisecond multiple=u32 200 ("millisecond timer value")) -> ()  [unwired: 1 out]
  }
  n230 = while {
    stop <- "stop 2" stop-if-true
    n231 = Current VI's Path() -> (path=w370:path)
    n232 = Path To String(path=w370) -> (string=w369:string)
    n233 = Match Pattern(string=w369, regular expression="\\.[Ee][Xx][Ee]") -> (offset past match=w367:i32)  [unwired: 1 in, 3 out]
    n234 = Equal?(x=w367, y=-1) -> (x = y?=w379:bool)
    n235 = case shown="True" w379 {
      tunnel: [w391 w393] -> w376
      tunnel: w370 -> [w392 w393]
      frame False {
        n236 = Strip Path(path=w392) -> (stripped path=w391:path)  [unwired: 1 out]
      }
      frame True {
      }
    }
    n237 = Path To String(path=w376) -> (string=w373:string)
    n238 = Match Pattern(string=w373, regular expression="\\.[Ll][Ll][Bb]") -> (offset past match=w375:i32)  [unwired: 1 in, 3 out]
    n239 = Equal?(x=w375, y=-1) -> (x = y?=w378:bool)
    n240 = case shown="True" w378 {
      tunnel: [w388 w390] -> w377
      tunnel: w376 -> [w389 w390]
      frame False {
        n241 = Strip Path(path=w389) -> (stripped path=w388:path)  [unwired: 1 out]
      }
      frame True {
      }
    }
    n242 = Strip Path(path=w377) -> (stripped path=w366:path)  [unwired: 1 out]
    n243 = Path To String(path=w366) -> (string=w365:string)
    n244 = Automation Open(Automation Refnum="WindowsMediaPlayer 3") -> (Automation Refnum=w382:refnum<k7>)  [unwired: 1 in, 3 out]
    n245 = Concatenate Strings(w365, "\\BMG.mp3" ("string")) -> (w386:string)
    n246 = property on="Property Node" class="IWMPPlayer4"(reference=w382, "URL"=w386) -> (reference out=w384:refnum<k7>, error out=w385:errorcluster)  [unwired: 1 in]
    n247 = Wait Until Next ms Multiple(millisecond multiple=u32 23000) -> ()  [unwired: 1 out]
    n248 = Close Reference(reference=w384, error in (no error)=w385) -> ()  [unwired: 1 out]
  }
